vi "StartSequenceAcquisition.vi"(8 "error in (no error)":errorcluster, 10 "DataExchange":T1, 11 "Stage_MadCityLab in":refnum<class "Stage_MadCityLab.lvclass">) -> (0 "error out":errorcluster, 3 "Stage_MadCityLab out":refnum<class "Stage_MadCityLab.lvclass">)   [LabVIEW 2020]
uses:
  Stage_MadCityLab.lvclass
  Hardware Abstraction Layer/Component/Device/Device/DeviceStatus.ctl
  Hardware Abstraction Layer/Component/Device/Device.lvlib
  Hardware Abstraction Layer/Component/Device/Device/DataExchange.ctl
  Interface/DataListener/DataListener.lvclass
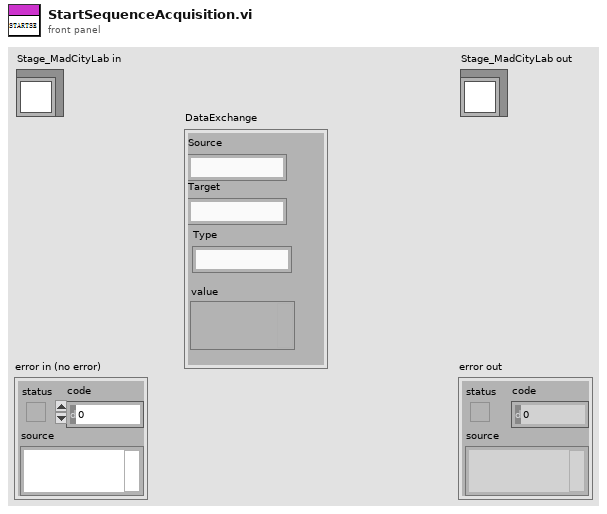
[diagram p1: front panel]
types:
  T1 = typedef "DataListener.lvclass/DataExchange.ctl" = cluster{"Source":string, "Target":string, "Type":string, "value":variant}
  T2 = typedef "Device.lvlib/DeviceStatus.ctl" = i32
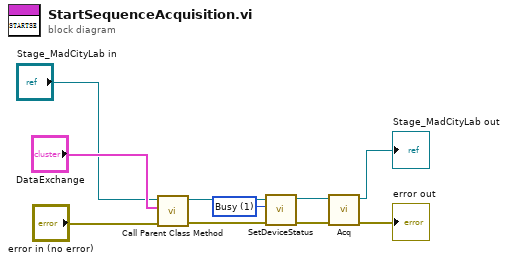
[diagram p0: block diagram]
diagram:
  w4 = T2 1 items=["Idle", "Busy"] ("Status")
  n1 = call-parent "Call Parent Class Method"("error in (no error)"="error in (no error)", "DataExchange"="DataExchange", "Device in"="Stage_MadCityLab in") -> ("error out"=w10:errorcluster, "Device out"=w5:refnum<class "Stage_MadCityLab.lvclass">)  [unwired: 7 in]
  n2 = call-dynamic "SetDeviceStatus.vi"("error in (no error)"=w10, "Status"=w4, "Device in"=w5) -> ("error out"=w6:errorcluster, "Device out"=w2:refnum<class "Stage_MadCityLab.lvclass">)  [unwired: 7 in]
  n3 = call-dynamic "Acq.vi"("error in (no error)"=w6, "Stage_MadCityLab in"=w2) -> ("error out"=→"error out":errorcluster, "Stage_MadCityLab out"=→"Stage_MadCityLab out":refnum<class "Stage_MadCityLab.lvclass">)  [unwired: 8 in]
